vi "S30c_dll wait.vi"(4 "error in (no error)":errorcluster caption="Fehlereingang", 5 "Time [ms]":u32=10) -> (0 "error out":errorcluster caption="Fehlerausgang")   [LabVIEW 2014, in "K_S30c_dll.lvlib"]
uses:
  K_S30c_dll.lvlib
panel:
  # "Wait if nor error"
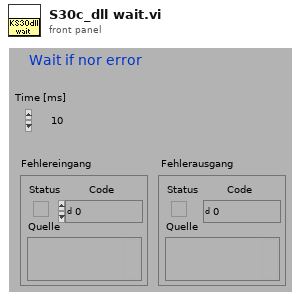
[diagram p1: front panel]
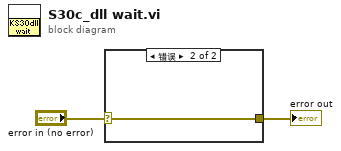
[diagram p0: block diagram]
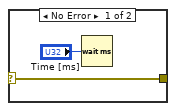
[diagram p2: hidden frame]
diagram:
  n1 = case shown="错误" "error in (no error)" {
    selector: "error in (no error)" -> [w3 w5]
    tunnel: [w3 w5] -> w1
    frame No Error {
      n2 = Wait (ms)(milliseconds to wait="Time [ms]") -> ()  [unwired: 1 out]
    }
    frame Error {
    }
  }
  "error out" <- w1
